vi "Charging_Extract VBAT Status from String.vi"(11 "Get VBAT String":string="VBAT     4095") -> (2 "VBAT (volts)":dbl=nan format="%.4f", 3 "ADC Counts":dbl=nan)   [LabVIEW 2020]
doc: "This function converts a string containg the IPG VBAT ADC count into volts.\n\nThe IPG VBAT ADC is 12-bit unsigned, full scale is 5.00 volts.\nThe ADC scale factor is 0.001221001 per ADC bit. (4095 * 0.001221001 = 5.0000 volts)"
panel:
  in  "LSB scale factor (constant)":dbl=0.001221001 format="%.9f"
  # "12-bit ADC unsigned, full scale = 5.00 volts"
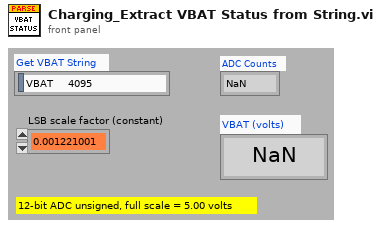
[diagram p1: front panel]
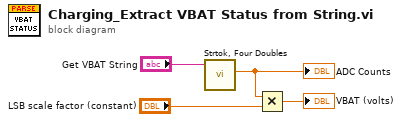
[diagram p0: block diagram]
diagram:
  n1 = call "Strtok, Four Doubles.vi"("input string"="Get VBAT String") -> ("x 2"=w1:dbl)  [unwired: 2 in, 3 out]
  "ADC Counts" <- w1
  n2 = Multiply(x=w1, y="LSB scale factor (constant)") -> (x*y=→"VBAT (volts)":dbl)
